vi "sub_calc-attractive_potential.vi"(10 "goal pt":cluster{"x":dbl, "y":dbl}, 11 "xy pt":cluster{"x":dbl, "y":dbl}) -> (3 "length":dbl)   [LabVIEW 2019]
uses:
  Ctrl/cmd_common.ctl
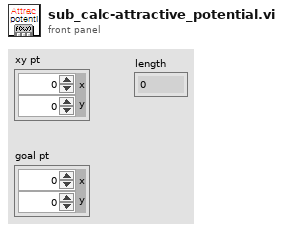
[diagram p1: front panel]
types:
  T1 = typedef "cmd_common.ctl" = enum16{"read", "write"}
  T2 = cluster{"KP":dbl, "ETA":dbl, "AREA_WIDTH":dbl, "Osc_Det_Len":u32}
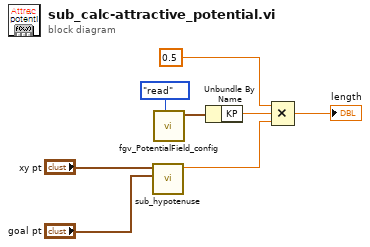
[diagram p0: block diagram]
diagram:
  n1 = call "sub_hypotenuse.vi"("x2y2"="goal pt", "x1y1"="xy pt") -> ("length"=w4:dbl)  [unwired: 9 in]
  n2 = call "fgv_PotentialField_config.vi"("cmd"=cmd_common."read") -> ("pf-val out"=w5:T2)  [unwired: 10 in]
  n3 = Unbundle By Name(w5) -> ("KP"=w3:dbl)
  n4 = Compound Arithmetic op=MULTIPLY(0.5 ("value"), w3, w4) -> (→"length":dbl)
